vi "Check_Traverse_move_Low.vi"(3 "Traverse Name":string, 4 "Probe Support XYZ?":bool, 5 "Exclude Array":T2[](array[typedef])=[{"Sizes"=[{"Max"=15000.0, "Min"=0.0}, {"Max"=1000.0, "Min"=-1000.0}, {"Max"=300.0, "Min"=0.0}], "Name"="Roughness Elements", "Exclude Type"=enum."Allow only vertical moves"}, {"Sizes"=[{"Max"=17000.0, "Min"=16000.0}, {"Max"=200.0, "Min"=-200.0}, {"Max"=-50.0, "Min"=-250.0}], "Name"="B204", "Exclude Type"=enum."Exclude completely"}] {"Sizes"."Min" format="%#.1f"; "Sizes"."Max" format="%#.1f"}, 6 "Probe Support":T1=[{"Max"=15001.0, "Min"=12000.0}, {"Max"=1000.0, "Min"=-1000.0}, {"Max"=700.0, "Min"=0.0}] {"Min" format="%#.1f"; "Max" format="%#.1f"}, 7 "Probe Volume":T1=[{"Max"=15.0, "Min"=-15.0}, {"Max"=250.0, "Min"=0.0}, {"Max"=15.0, "Min"=-15.0}] {"Min" format="%#.1f"; "Max" format="%#.1f"}, 8 "New Position":sgl[](array[numeric])=[0.0, 0.0, 0.0] format="%.2f", 9 "Current position":sgl[](array[numeric])=[0.0, 0.0, 0.0] format="%.2f") -> (0 "Error Comments":string, 2 "Position At Crash":dbl[](array[numeric]) format="%.2f")   [LabVIEW 2018]
uses:
  Box_size.ctl
  Exclude_cluster.ctl
  Exclusion_type.ctl
  Globals/Trav_pos_global.vi
panel:
  out "Numeric":i32
  # "X                Y                   Z"
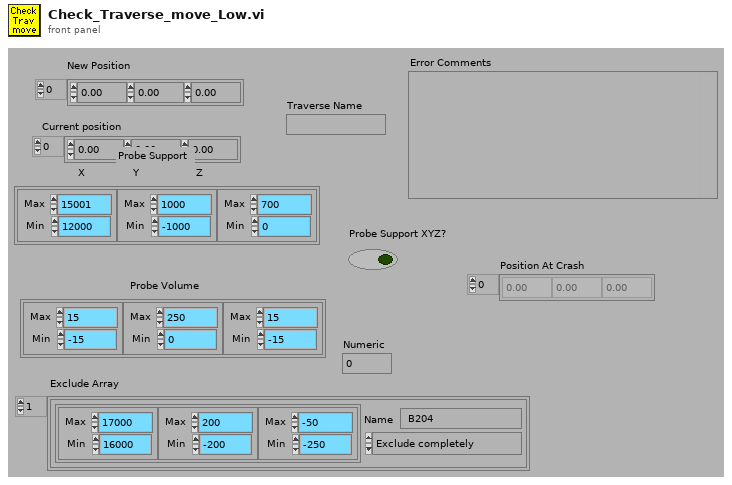
[diagram p1: front panel]
types:
  T1 = typedef "Box_size.ctl" = cluster{"Max":sgl, "Min":sgl}[]
  T2 = typedef "Exclude_cluster.ctl" = cluster{"Sizes":T1, "Name":string, "Exclude Type":T3}
  T3 = typedef "Exclusion_type.ctl" = enum16{"Exclude completely", "Allow only vertical moves"}
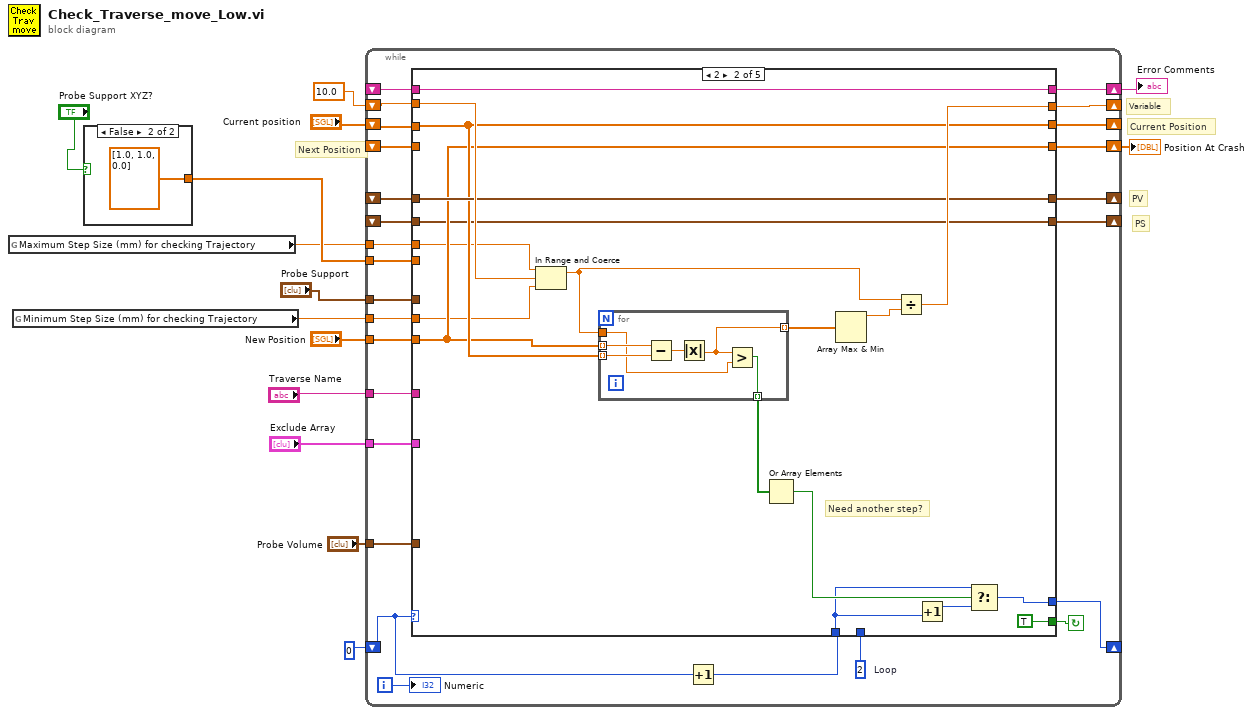
[diagram p0: block diagram]
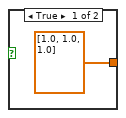
[diagram p2: hidden frame]
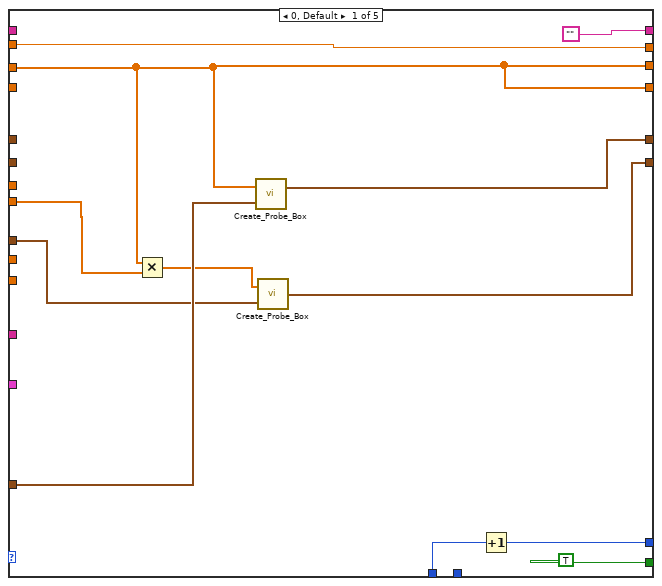
[diagram p3: hidden frame]
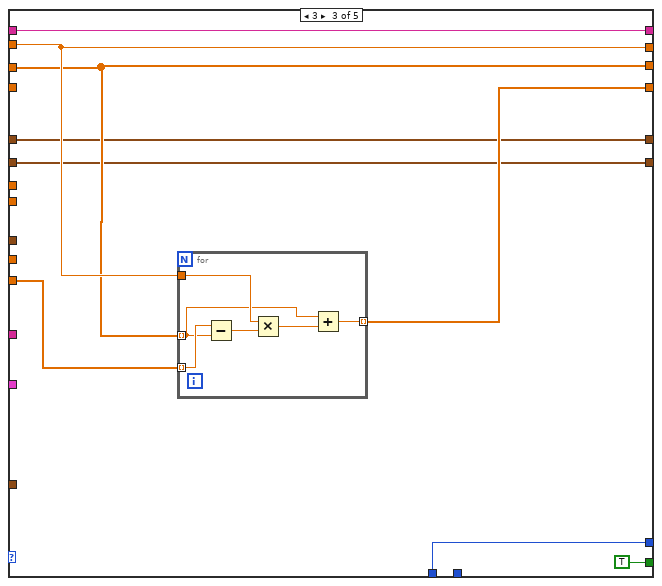
[diagram p4: hidden frame]
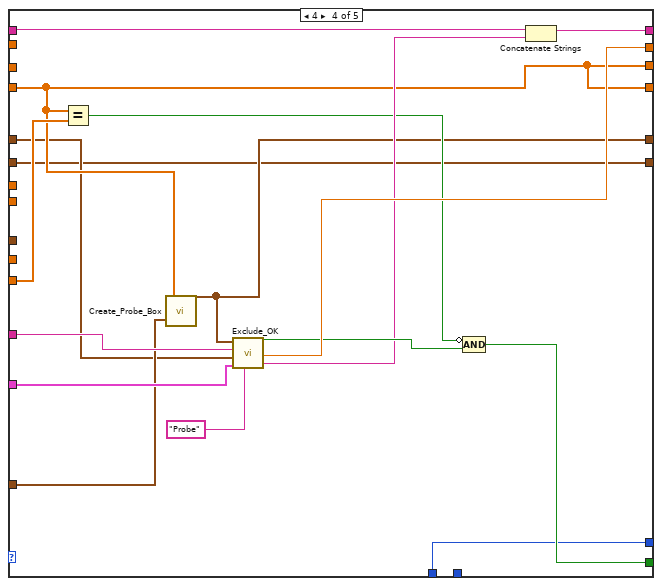
[diagram p5: hidden frame]
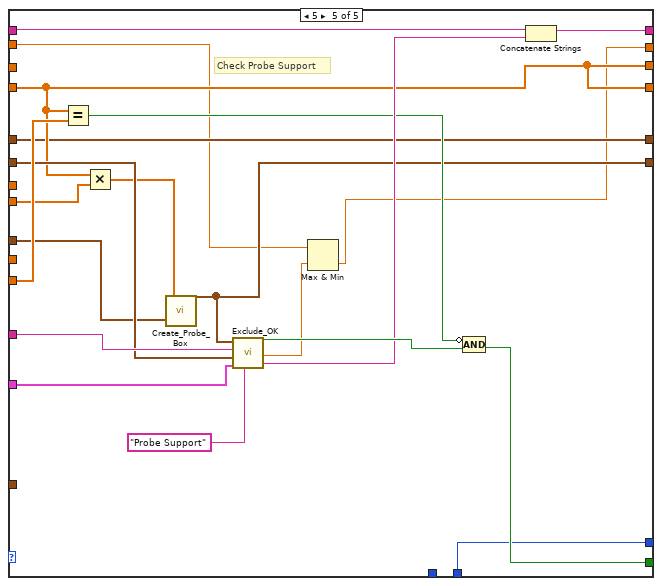
[diagram p6: hidden frame]
diagram:
  # "PS"
  # "PV"
  # "Current Position"
  # "Next Position"
  # "Variable"
  n1 = global read "Trav_pos_global.vi" "Maximum Step Size (mm) for checking Trajectory"() -> (w3:sgl)
  n2 = global read "Trav_pos_global.vi" "Minimum Step Size (mm) for checking Trajectory"() -> (w1:sgl)
  n3 = case shown="False" "Probe Support XYZ?" {
    tunnel: [sgl[] [1.0, 1.0, 1.0] ("Current position") sgl[] [1.0, 1.0, 0.0] ("Current position")] -> w4
    frame True {
    }
    frame False {
    }
  }
  n4 = while {
    shift-left: _ -> [w23]
    shift-right: [w24] -> _
    tunnel: "Probe Volume" -> [w26]
    tunnel: "New Position" -> [w28]
    shift-left: _ -> [w30]
    shift-right: [w31] -> w10
    shift-left: 0 -> [w34]
    shift-right: [w33] -> _
    tunnel: "Traverse Name" -> [w35]
    tunnel: "Exclude Array" -> [w37]
    shift-left: sgl 10.0 ("Separation Distance") -> [w41]
    shift-right: [w36] -> _
    shift-left: _ -> [w29]
    shift-right: [w39] -> w8
    shift-left: "Current position" -> [w42]
    shift-right: [w40] -> _
    shift-right: [w21] -> _
    shift-left: _ -> [w20]
    tunnel: "Probe Support" -> [w22]
    tunnel: w4 -> [w19]
    tunnel: w3 -> [w18]
    tunnel: w1 -> [w17]
    i -> [w25]
    stop <- w38 continue-if-true
    w27 = 2  # Loop
    n5 = Increment(x=w34) -> (x+1=w32:i32)
    n6 = case shown="2" w34 {
      tunnel: w42 -> [w44 w60 w84 _ _]
      tunnel: w41 -> [w54 w72 w85 _ w113]
      tunnel: [w44 w60 w84 w101 w119] -> w40
      tunnel: [w44 w59 w83 w101 w119] -> w39
      tunnel: [TRUE ("Box Inside") TRUE ("Box Inside") TRUE ("Box Inside") w97 w123] -> w38
      tunnel: w26 -> [w52 _ _ w100 _]
      tunnel: w37 -> [_ _ _ w110 w131]
      tunnel: [w54 w66 w85 w109 w111] -> w36
      tunnel: w35 -> [_ _ _ w108 w130]
      tunnel: [w48 w64 w81 w96 w122] -> w33
      tunnel: w32 -> [w51 w62 w81 w96 _]
      tunnel: ["" w70 w87 w105 w127] -> w31
      tunnel: w30 -> [_ w70 w87 w106 w128]
      tunnel: w29 -> [_ _ _ w101 w119]
      tunnel: w28 -> [_ w59 w82 w103 w125]
      tunnel: w27 -> [_ _ _ _ w122]
      tunnel: [w49 w61 w80 w99 w115] -> w24
      tunnel: w23 -> [_ w61 w80 w98 w115]
      tunnel: w22 -> [w47 _ _ _ w120]
      tunnel: [w46 w57 w79 w95 w116] -> w21
      tunnel: w20 -> [_ w57 w79 w95 w121]
      tunnel: w19 -> [w45 _ _ _ w118]
      tunnel: w18 -> [_ w56 _ _ _]
      tunnel: w17 -> [_ w55 _ _ _]
      frame 0, Default {
        n7 = Multiply(x=w44, y=w45) -> (x*y=w43:sgl[])
        n8 = call "Create_Probe_Box.vi"("Probe Volume"=w52, "Probe Position"=w44) -> ("Current Probe Volume"=w49:T1)
        n9 = call "Create_Probe_Box.vi"("Probe Volume"=w47, "Probe Position"=w43) -> ("Current Probe Volume"=w46:T1)
        n10 = Increment(x=w51) -> (x+1=w48:i32)
      }
      frame 2 {
        # "Need another step?"
        n11 = In Range and Coerce(upper limit=w56, x=w72, lower limit=w55) -> (coerced(x)=w58:sgl)  [unwired: 1 out]
        n12 = for {
          tunnel: w59 -> [w78] mode=indexing
          tunnel: w60 -> [w77] mode=indexing
          tunnel: w58 -> [w76]
          tunnel: [w74] -> w69 mode=indexing
          tunnel: [w73] -> w68 mode=indexing
          n13 = Subtract(x=w78, y=w77) -> (x-y=w75:sgl)
          n14 = Absolute Value(x=w75) -> (abs(x)=w73:sgl)
          n15 = Greater?(x=w73, y=w76) -> (0:w74:bool)
        }
        n16 = Or Array Elements(Boolean array=w69) -> (logical OR=w65:bool)
        n17 = Array Max & Min(array=w68) -> (max value=w67:sgl)  [unwired: 3 out]
        n18 = Divide(x=w58, y=w67) -> (x/y=w66:sgl)
        n19 = Increment(x=w62) -> (x+1=w63:i32)
        n20 = Select(t=w62, s=w65, f=w63) -> (s? t:f=w64:i32)
      }
      frame 3 {
        n21 = for {
          tunnel: w82 -> [w93] mode=indexing
          tunnel: w84 -> [w89] mode=indexing
          tunnel: w85 -> [w91]
          tunnel: [w88] -> w83 mode=indexing
          n22 = Subtract(x=w93, y=w89) -> (x-y=w92:sgl)
          n23 = Multiply(x=w91, y=w92) -> (x*y=w90:sgl)
          n24 = Add(x=w89, y=w90) -> (x+y=w88:sgl)
        }
      }
      frame 4 {
        n25 = Equal?(x=w101, y=w103) -> (x = y?=w102:bool)
        n26 = call "Create_Probe_Box.vi"("Probe Volume"=w100, "Probe Position"=w101) -> ("Current Probe Volume"=w99:T1)
        n27 = call "Exclude_OK.vi"("Probe Volume"=w99, "Traverse Name"=w108, "Previous Probe Volume"=w98, "Exclude Array"=w110, "Volume Name"="Probe") -> ("Probe OK?"=w107:bool, "Separation Distance"=w109:sgl, "Error Comments"=w104:string)
        n28 = Compound Arithmetic op=AND(invert w102, w107) -> (w97:bool)
        n29 = Concatenate Strings(w106, w104) -> (w105:string)
      }
      frame 5 {
        # "Check Probe Support"
        n30 = Equal?(x=w119, y=w125) -> (x = y?=w124:bool)
        n31 = Multiply(x=w119, y=w118) -> (x*y=w117:sgl[])
        n32 = call "Create_Probe_Box.vi"("Probe Volume"=w120, "Probe Position"=w117) -> ("Current Probe Volume"=w116:T1)
        n33 = call "Exclude_OK.vi"("Probe Volume"=w116, "Traverse Name"=w130, "Previous Probe Volume"=w121, "Exclude Array"=w131, "Volume Name"="Probe Support") -> ("Probe OK?"=w129:bool, "Separation Distance"=w112:sgl, "Error Comments"=w126:string)
        n34 = Max & Min(x=w113, y=w112) -> (min(x,y)=w111:sgl)  [unwired: 1 out]
        n35 = Compound Arithmetic op=AND(invert w124, w129) -> (w123:bool)
        n36 = Concatenate Strings(w128, w126) -> (w127:string)
      }
    }
    "Numeric" <- w25
  }
  "Error Comments" <- w10
  "Position At Crash" <- w8
